vi "SHT20.vi"() -> ()   [LabVIEW 2024]
uses:
  <vilib>/MakerHub/LINX/Public/Utilities/Open Local.vi
  <vilib>/MakerHub/LINX/LMH-LINX.lvlib
panel:
  out "RH":dbl
  out "Temperature":dbl
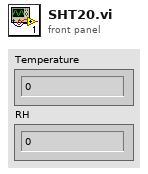
[diagram p1: front panel]
types:
  T1 = cluster{"I2C Slave Address":u8, "T Offset":dbl, "RH Offset":dbl, "I2C Channel":u8}
  T2 = typedef "LMH-LINX.lvlib/LINX Ref.ctl" = cluster{"IO":T3, "Interface":T4, "LINX Device Config":T5}
  T3 = typedef "LMH-LINX.lvlib/Platform.ctl" = enum16{"Remote", "Local"}
  T4 = typedef "LMH-LINX.lvlib/Interface.ctl" = enum16{"Serial", "TCP"}
  T5 = typedef "LMH-LINX.lvlib/Device.lvlib/LINX Device Config.ctl" = cluster{"Interface":T4, "COM Port":refnum<visa-resource-name>, "TCP Configuration":T6, "Device Family":u8, "Device ID":u8, "Device Name":string, "TCP Ref":refnum<k5>, "Channels":T7}
  T6 = typedef "LMH-LINX.lvlib/Device.lvlib/TCP Config.ctl" = cluster{"IP Address":string, "Port":u16}
  T7 = typedef "LMH-LINX.lvlib/Channels.ctl" = cluster{"DI":u8[], "DO":u8[], "AI":u8[], "AO":u8[], "PWM":u8[], "QE":u8[], "UART":u8[], "I2C 2":u8[], "SPI":u8[], "CAN":u8[], "Servo":u8[], "AI Ref (V)":dbl, "AI Resolution (Bits)":u8, "AO Ref (V)":dbl, "AO Resolution (Bits)":u8}
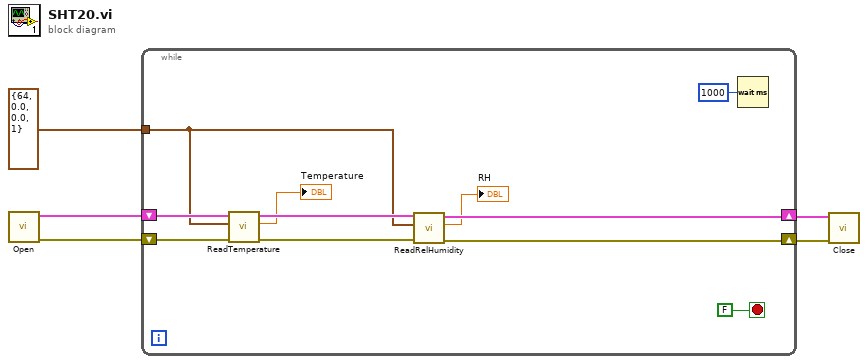
[diagram p0: block diagram]
diagram:
  n1 = call-poly <vilib>:"Open.vi"() -> ("Error Out"=w4:errorcluster, "LINX Resource"=w5:T2)  [unwired: 9 in, 1 out]
  n2 = while {
    tunnel: T1 {"I2C Slave Address"=64, "T Offset"=0.0, "RH Offset"=0.0, "I2C Channel"=1} ("Cluster") -> [w7]
    shift-right: [w11] -> w3
    shift-left: w5 -> [w15]
    shift-right: [w10] -> w2
    shift-left: w4 -> [w14]
    stop <- FALSE stop-if-true
    n3 = call "ReadTemperature.vi"("Error In"=w14, "Cluster"=w7, "LINX Resource"=w15) -> ("Error Out"=w12:errorcluster, "Temperature"=→"Temperature":dbl, "LINX Resource"=w13:T2)  [unwired: 4 in]
    n4 = call "ReadRelHumidity.vi"("Error In"=w12, "Cluster"=w7, "LINX Resource"=w13) -> ("Error Out"=w10:errorcluster, "RH"=→"RH":dbl, "LINX Resource"=w11:T2)  [unwired: 3 in, 1 out]
    n5 = Wait (ms)(milliseconds to wait=u32 1000) -> ()  [unwired: 1 out]
  }
  n6 = call <vilib>:"Close.vi"("Error In"=w2, "LINX Resource"=w3) -> ()  [unwired: 9 in, 1 out]
